vi "Write useTerminate.vi"(8 "error in (no error)":errorcluster, 10 "useTerminate":bool=TRUE, 11 "Orion_BMS in":refnum<class "Orion_BMS.lvclass">) -> (0 "error out":errorcluster, 3 "Orion_BMS out":refnum<class "Orion_BMS.lvclass">)   [LabVIEW 2017, in "Orion_BMS.lvclass"]
uses:
  Orion_BMS.lvclass
  Orion_BMS.lvclass/Orion_BMS.ctl
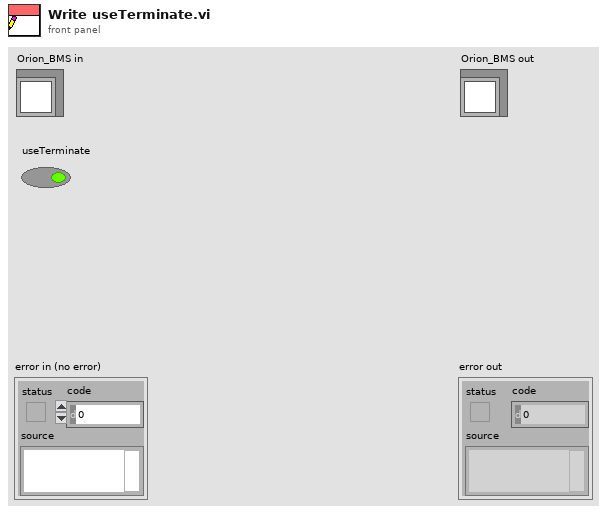
[diagram p1: front panel]
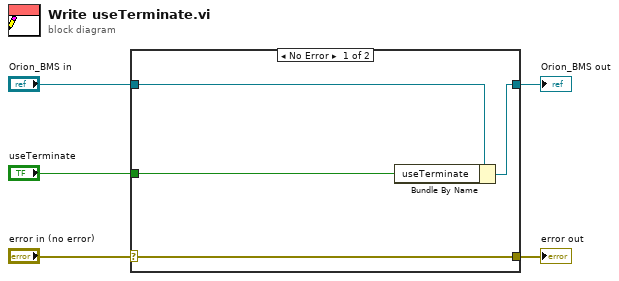
[diagram p0: block diagram]
diagram:
  n1 = case shown="No Error" "error in (no error)" {
    selector: "error in (no error)" -> [w9 w10]
    tunnel: [w9 w10] -> w4
    tunnel: [w7 w11] -> w2
    tunnel: "Orion_BMS in" -> [w8 w11]
    tunnel: "useTerminate" -> [w6 _]
    frame No Error {
      n2 = Bundle By Name(cluster=w8, "useTerminate"=w6) -> (w7:refnum<class "Orion_BMS.lvclass">)
    }
    frame Error {
    }
  }
  "error out" <- w4
  "Orion_BMS out" <- w2
